vi "execute_command.vi"(8 "error in (no error)":errorcluster, 11 "canon_m3 in":refnum<class "canon_m3.lvclass">) -> (0 "error out":errorcluster, 3 "canon_m3 out":refnum<class "canon_m3.lvclass">)   [LabVIEW 2015, in "canon_m3.lvclass"]
uses:
  canon_m3.lvclass
  canon_m3.lvclass/canon_m3.ctl
panel:
  out "MessageLog":string[](array[string])
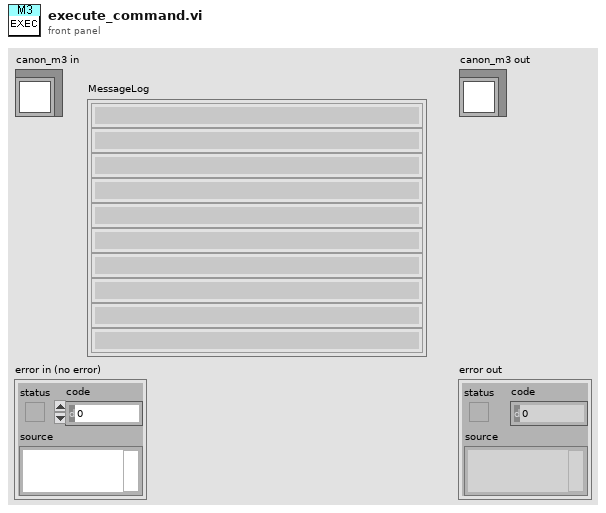
[diagram p1: front panel]
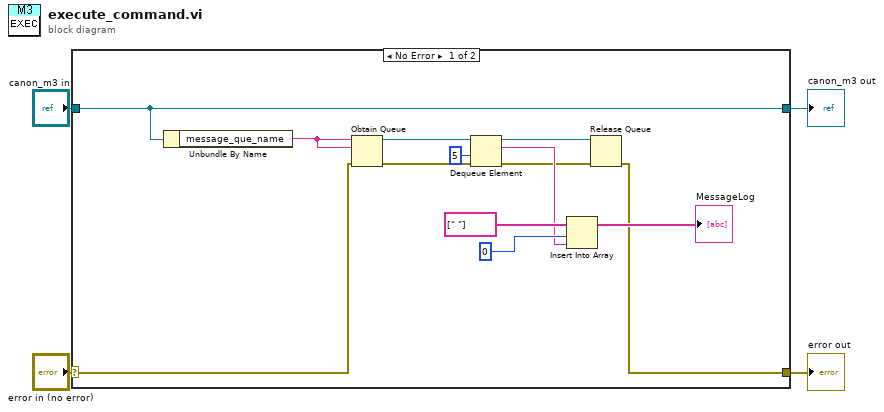
[diagram p0: block diagram]
diagram:
  n1 = case shown="No Error" "error in (no error)" {
    selector: "error in (no error)" -> [w7 w19]
    tunnel: [w6 w19] -> w3
    tunnel: [w11 w18] -> w1
    tunnel: "canon_m3 in" -> [w11 w18]
    frame No Error {
      n2 = Unbundle By Name(w11) -> ("message_que_name"=w10:string)
      n3 = Obtain Queue(name (unnamed)=w10, element data type=w10, error in (no error)=w7) -> (queue out=w17:refnum<queue>, error out=w9:errorcluster)  [unwired: 2 in, 1 out]
      n4 = Dequeue Element(queue=w17, timeout in ms (-1)=5, error in (no error)=w9) -> (queue out=w12:refnum<queue>, element=w14:string, error out=w8:errorcluster)  [unwired: 1 out]
      n5 = Insert Into Array(array=string[] [" "] ("Array"), index=0, new element=w14) -> (→"MessageLog":string[])
      n6 = Release Queue(queue=w12, error in (no error)=w8) -> (error out=w6:errorcluster)  [unwired: 1 in, 2 out]
    }
    frame Error {
    }
  }
  "error out" <- w3
  "canon_m3 out" <- w1
